vi "Go Home SubVi.vi"(2 "error in":errorcluster, 3 "reference in":refnum<k24>) -> (0 "error out":errorcluster, 1 "reference out":refnum<k24>)   [LabVIEW 2017]
uses:
  Newport.XPS.CommandInterface
  Go Home Enum.ctl
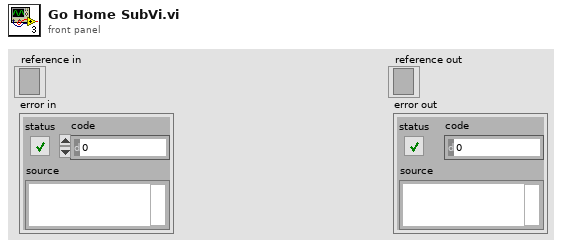
[diagram p1: front panel]
types:
  T1 = typedef "Go Home Enum.ctl" = enum16{"Change Velocity", "Go Home", "Stop Command"}
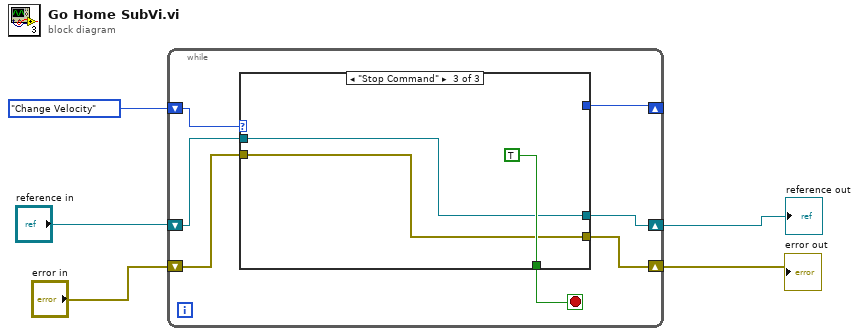
[diagram p0: block diagram]
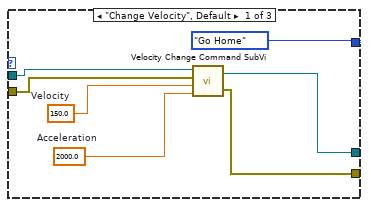
[diagram p2: hidden frame]
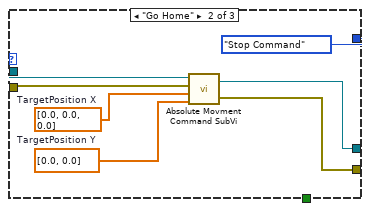
[diagram p3: hidden frame]
diagram:
  n1 = while {
    shift-right: [w7] -> _
    shift-left: Go_Home_Enum."Change Velocity" -> [w12]
    shift-right: [w8] -> w2
    shift-left: "error in" -> [w10]
    shift-right: [w9] -> w3
    shift-left: "reference in" -> [w11]
    stop <- w6 stop-if-true
    n2 = case shown="\"Stop Command\"" w12 {
      tunnel: w11 -> [w18 w25 w28]
      tunnel: w10 -> [w17 w24 w27]
      tunnel: [w14 w21 w28] -> w9
      tunnel: [w13 w20 w27] -> w8
      tunnel: [Go_Home_Enum."Go Home" Go_Home_Enum."Stop Command" _] -> w7
      tunnel: [_ _ TRUE] -> w6
      frame "Change Velocity", Default {
        w15 = 2000.0  # Acceleration
        w16 = 150.0  # Velocity
        n3 = call "Velocity Change Command SubVi.vi"("Acceleration"=w15, "Velocity"=w16, "error in"=w17, "reference in"=w18) -> ("error out"=w13:errorcluster, "reference out"=w14:refnum<k24>)
      }
      frame "Go Home" {
        w23 = dbl[] [0.0, 0.0]  # TargetPosition Y
        w22 = dbl[] [0.0, 0.0, 0.0]  # TargetPosition X
        n4 = call "Absolute Movment Command SubVi.vi"("TargetPosition Y"=w23, "TargetPosition X"=w22, "error in"=w24, "reference in"=w25) -> ("error out"=w20:errorcluster, "reference out"=w21:refnum<k24>)
      }
      frame "Stop Command" {
      }
    }
  }
  "reference out" <- w3
  "error out" <- w2
